vi "VALVE_init.vi"(3 "error in":errorcluster, 5 "VISA resource Valve":refnum<visa-resource-name>) -> (0 "error out":errorcluster, 1 "Error valve":bool, 2 "VISA resource name out":refnum<visa-resource-name>)   [LabVIEW 2015]
uses:
  <vilib>/Instr/_visa.llb/VISA Configure Serial Port (Instr).vi
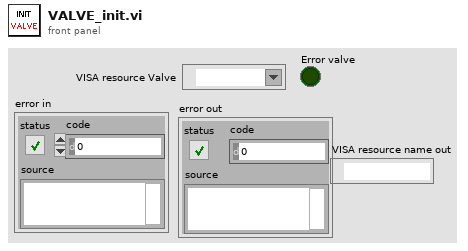
[diagram p1: front panel]
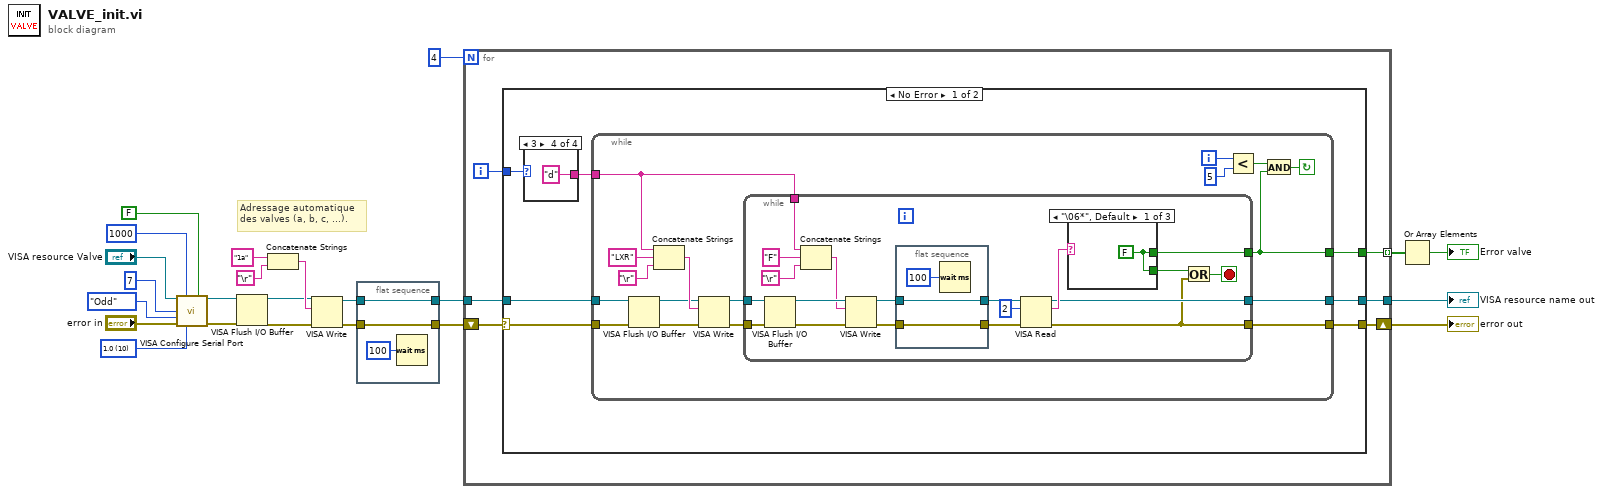
[diagram p0: block diagram]
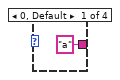
[diagram p2: hidden frame]
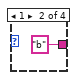
[diagram p3: hidden frame]
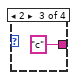
[diagram p4: hidden frame]
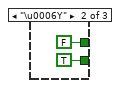
[diagram p5: hidden frame]
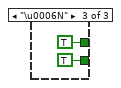
[diagram p6: hidden frame]
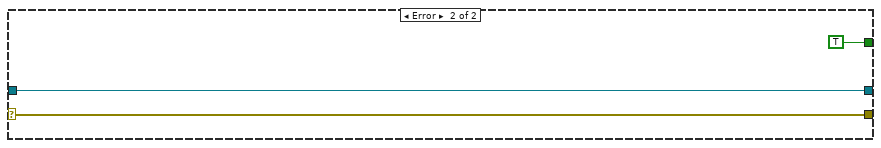
[diagram p7: hidden frame]
diagram:
  w14 = u16 10 items=["1.0"=10, "1.5"=15, "2.0"=20] ("stop bits (10: 1 bit)")
  # "Adressage automatique\ndes valves (a, b, c, ...)."
  n1 = call-poly "VISA Configure Serial Port"("VISA resource name"="VISA resource Valve", "timeout (10sec)"=u32 1000, "Enable Termination\nChar (T)"=FALSE ("Enable Termination\nChar (T)"), "data bits (8)"=u16 7, "parity (0:none)"=enum16{"None", "Odd", "Even", "Mark", "Space"}."Odd", "error in (no error)"="error in", "stop bits (10: 1 bit)"=w14) -> ("VISA resource name out"=w17:refnum<visa-resource-name>, "error out"=w16:errorcluster)  [unwired: 7 in]
  n2 = VISA Flush I/O Buffer(VISA resource name=w17, error in (no error)=w16) -> (VISA resource name out=w18:refnum<visa-resource-name>, error out=w19:errorcluster)  [unwired: 1 in]
  n3 = Concatenate Strings("1a" ("buffer d'écriture"), "\r") -> (w22:string)
  n4 = VISA Write(VISA resource name=w18, write buffer=w22, error in (no error)=w19) -> (VISA resource name out=w11:refnum<visa-resource-name>, error out=w9:errorcluster)  [unwired: 1 out]
  n5 = flat-sequence {
    tunnel: w11 -> [w26]
    tunnel: [w26] -> w10
    tunnel: w9 -> [w25]
    tunnel: [w25] -> w4
    frame #0 {
      n6 = Wait (ms)(milliseconds to wait=u32 100) -> ()  [unwired: 1 out]
    }
  }
  n7 = for {
    N: 4 -> [_]
    tunnel: w10 -> [w32]
    tunnel: [w30] -> w1 mode=indexing
    tunnel: [w29] -> w5
    shift-right: [w28] -> w7
    shift-left: w4 -> [w27]
    i -> [w31]
    n8 = case shown="No Error" w27 {
      selector: w27 -> [w33 w90]
      tunnel: w32 -> [w39 w89]
      tunnel: w31 -> [w38 _]
      tunnel: [w36 TRUE] -> w30
      tunnel: [w35 w89] -> w29
      tunnel: [w34 w90] -> w28
      frame No Error {
        n9 = case shown="3" w38 {
          tunnel: ["a" "b" "c" "d"] -> w37
          frame 0, Default {
          }
          frame 1 {
          }
          frame 2 {
          }
          frame 3 {
          }
        }
        n10 = while {
          tunnel: w33 -> [w50]
          tunnel: [w58] -> w34
          tunnel: w39 -> [w60]
          tunnel: [w59] -> w35
          tunnel: [w45] -> w36
          tunnel: w37 -> [w44]
          i -> [w49]
          stop <- w46 continue-if-true
          n11 = VISA Flush I/O Buffer(VISA resource name=w60, error in (no error)=w50) -> (VISA resource name out=w54:refnum<visa-resource-name>, error out=w55:errorcluster)  [unwired: 1 in]
          n12 = Concatenate Strings(w44, "LXR" ("string"), "\r") -> (w57:string)
          n13 = VISA Write(VISA resource name=w54, write buffer=w57, error in (no error)=w55) -> (VISA resource name out=w52:refnum<visa-resource-name>, error out=w51:errorcluster)  [unwired: 1 out]
          n14 = while {
            tunnel: w51 -> [w73]
            tunnel: w52 -> [w72]
            tunnel: [w61] -> w58
            tunnel: [w66] -> w59
            tunnel: [w65] -> w45
            tunnel: w44 -> [w64]
            stop <- w63 stop-if-true
            n15 = VISA Flush I/O Buffer(VISA resource name=w72, error in (no error)=w73) -> (VISA resource name out=w71:refnum<visa-resource-name>, error out=w70:errorcluster)  [unwired: 1 in]
            n16 = Concatenate Strings(w64, "F" ("string"), "\r") -> (w68:string)
            n17 = VISA Write(VISA resource name=w71, write buffer=w68, error in (no error)=w70) -> (VISA resource name out=w75:refnum<visa-resource-name>, error out=w76:errorcluster)  [unwired: 1 out]
            n18 = flat-sequence {
              tunnel: w75 -> [w87]
              tunnel: [w87] -> w77
              tunnel: w76 -> [w86]
              tunnel: [w86] -> w78
              frame #0 {
                n19 = Wait (ms)(milliseconds to wait=u32 100) -> ()  [unwired: 1 out]
              }
            }
            n20 = VISA Read(VISA resource name=w77, byte count=u32 2, error in (no error)=w78) -> (VISA resource name out=w66:refnum<visa-resource-name>, read buffer=w67:string, error out=w61:errorcluster)  [unwired: 1 out]
            n21 = case shown="\"\\06*\", Default" w67 {
              tunnel: [w80 FALSE TRUE] -> w65
              tunnel: [w80 TRUE TRUE] -> w62
              frame "\u0006*", Default {
                w80 = FALSE
              }
              frame "\u0006Y" {
              }
              frame "\u0006N" {
              }
            }
            n22 = Or(x=w62, y=w61) -> (x .or. y?=w63:bool)
          }
          n23 = Less?(x=w49, y=5) -> (x < y?=w47:bool)
          n24 = And(x=w47, y=w45) -> (x .and. y?=w46:bool)
        }
      }
      frame Error {
      }
    }
  }
  "error out" <- w7
  "VISA resource name out" <- w5
  n25 = Or Array Elements(Boolean array=w1) -> (logical OR=→"Error valve":bool)
